vi "GetAllSerialComm.vi"(0 "VISA Address":string, 1 "reference":refnum<vi>) -> (2 "List":string[](array[string]), 3 "new?":bool, 4 "names":string[](array[string]))   [LabVIEW 2014]
panel:
  out "Array":string[](array[string])
  out "find list":string[](array[string])
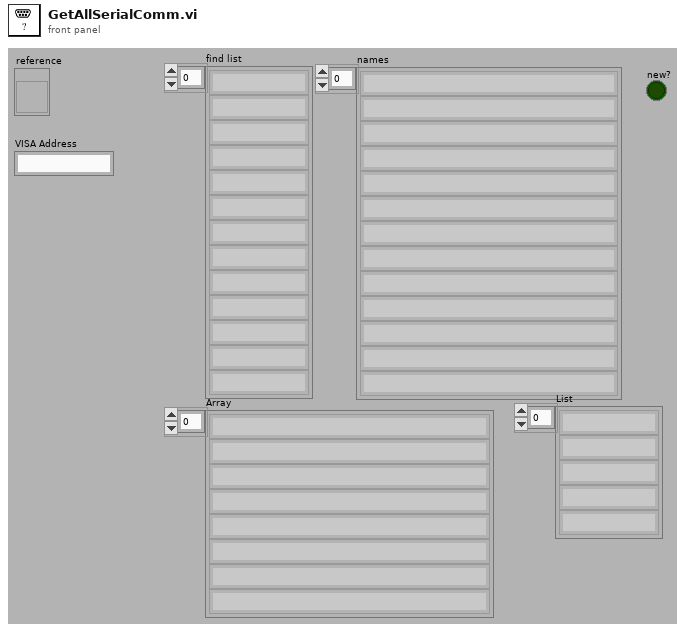
[diagram p1: front panel]
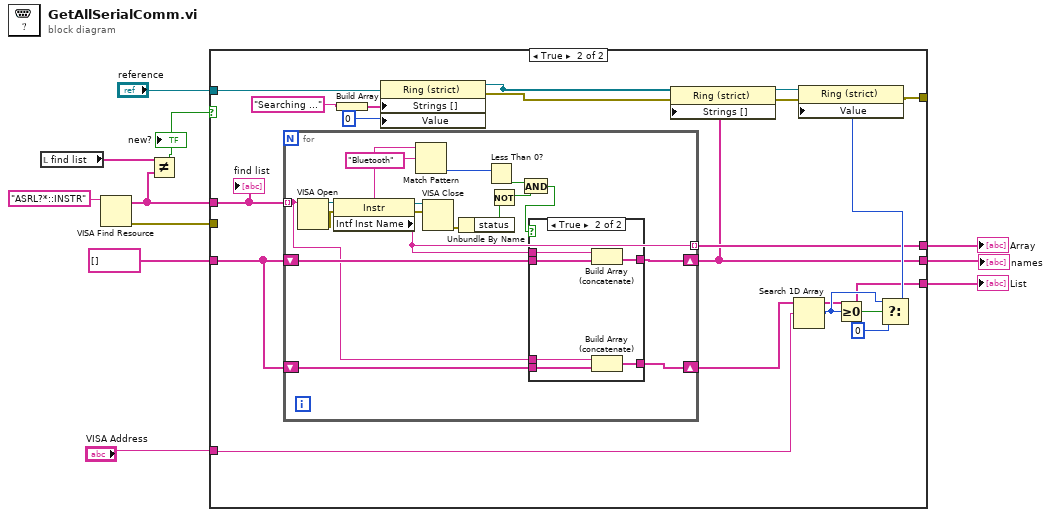
[diagram p0: block diagram]
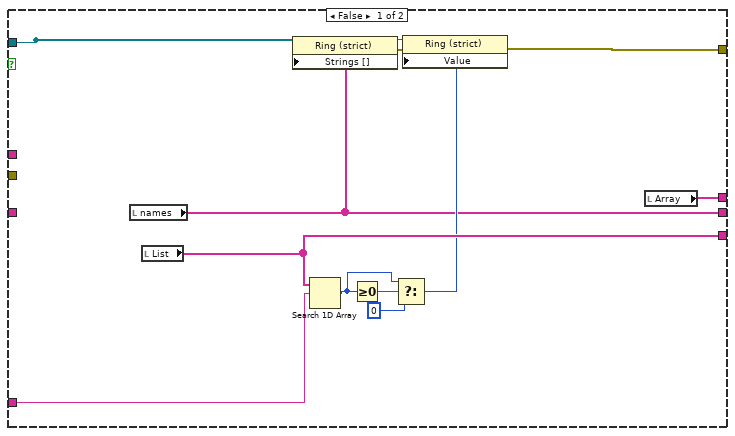
[diagram p2: hidden frame]
diagram:
  n1 = local read "find list"() -> (w6:string[])
  n2 = VISA Find Resource(11:"ASRL?*::INSTR" ("expression (\"?*\")")) -> (0:w2:errorcluster, 3:w7:string[])  [unwired: 2 in, 1 out]
  n3 = Not Equal?(x=w6, y=w7) -> (x != y?=w1:bool)
  "new?" <- w1
  n4 = case shown="True" w1 {
    tunnel: string[] [] -> [_ w36]
    tunnel: "VISA Address" -> [w14 w35]
    tunnel: "reference" -> [w20 w25]
    tunnel: [w19 w33] -> _
    tunnel: w7 -> [_ w32]
    tunnel: [w22 w31] -> w5
    tunnel: [w12 w30] -> w4
    tunnel: [w15 w29] -> w3
    tunnel: w2 -> [_ _]
    frame False {
      n5 = local read "names"() -> (w12:string[])
      n6 = local read "List"() -> (w15:string[])
      n7 = property on="Property Node" class="Ring (strict)"(reference=w20, "Strings []"=w12) -> (error out=w21:errorcluster)  [unwired: 1 in, 1 out]
      n8 = Search 1D Array(1D array=w15, element=w14) -> (index of element=w17:i32)  [unwired: 1 in]
      n9 = Greater Or Equal To 0?(x=w17) -> (x >= 0?=w16:bool)
      n10 = Select(t=w17, s=w16, f=0) -> (s? t:f=w13:i32)
      n11 = property class="Ring (strict)"(reference=w20, error in=w21, "Value"=w13) -> (error out=w19:errorcluster)  [unwired: 1 out]
      n12 = local read "Array"() -> (w22:string[])
    }
    frame True {
      n13 = for {
        tunnel: w32 -> [w50] mode=indexing
        shift-right: [w53] -> w30
        shift-left: w36 -> [w52]
        tunnel: [w48] -> w31 mode=indexing
        shift-right: [w51] -> w29
        shift-left: w36 -> [w49]
        n14 = VISA Open(VISA resource name=w50) -> (VISA resource name=w57:refnum<visa-resource-name>, error out=w55:errorcluster)  [unwired: 4 in]
        n15 = property class="Instr"(reference=w57, error in=w55) -> (reference out=w56:refnum<visa-resource-name>, error out=w54:errorcluster, "Intf Inst Name"=w48:string)
        n16 = Match Pattern(string=w48, regular expression="Bluetooth" ("task")) -> (offset past match=w46:i32)  [unwired: 1 in, 3 out]
        n17 = VISA Close(VISA resource name=w56, error in (no error)=w54) -> (error out=w44:errorcluster)
        n18 = Unbundle By Name(w44) -> ("status"=w43:bool)
        n19 = Less Than 0?(x=w46) -> (x < 0?=w45:bool)
        n20 = Not(x=w43) -> (.not. x?=w42:bool)
        n21 = And(x=w45, y=w42) -> (x .and. y?=w41:bool)
        n22 = case shown="True" w41 {
          tunnel: w48 -> [_ w60]
          tunnel: [w59 w65] -> w53
          tunnel: w52 -> [w59 w64]
          tunnel: [w58 w63] -> w51
          tunnel: w50 -> [_ w62]
          tunnel: w49 -> [w58 w61]
          frame False {
          }
          frame True {
            n23 = Build Array (concatenate)(w60, w64) -> (w65:string[])
            n24 = Build Array (concatenate)(w62, w61) -> (w63:string[])
          }
        }
      }
      n25 = Build Array("Searching ..." ("task")) -> (w27:string[])
      n26 = property on="Property Node" class="Ring (strict)"(reference=w25, "Strings []"=w27, "Value"=0) -> (reference out=w24:refnum<vi>, error out=w23:errorcluster)  [unwired: 1 in]
      n27 = property on="Property Node" class="Ring (strict)"(reference=w24, error in=w23, "Strings []"=w30) -> (error out=w34:errorcluster)  [unwired: 1 out]
      n28 = Search 1D Array(1D array=w29, element=w35) -> (index of element=w38:i32)  [unwired: 1 in]
      n29 = Greater Or Equal To 0?(x=w38) -> (x >= 0?=w37:bool)
      n30 = Select(t=w38, s=w37, f=0) -> (s? t:f=w40:i32)
      n31 = property class="Ring (strict)"(reference=w24, error in=w34, "Value"=w40) -> (error out=w33:errorcluster)  [unwired: 1 out]
      "find list" <- w32
    }
  }
  "Array" <- w5
  "names" <- w4
  "List" <- w3
